vi "LV8_3.vi"() -> ()   [LabVIEW 2016]
uses:
  <vilib>/sound2/lvsound2.llb/Sampling Mode.ctl
  <vilib>/Utility/file.llb/Read From Spreadsheet File (DBL).vi
  <vilib>/imath/engines/lvmath2/RunTimeEngine/BuiltInFunctions/length/NIMS_length(GV).vi
  <instcachedir>/0/NIMS_length(GV)_08A3D13377FD4E4B96F5795FBF3698FA.lvgen/NIMS_length(GV)_08A3D13377FD4E4B96F5795FBF3698FA_000.vi
  <vilib>/imath/engines/lvmath2/RunTimeEngine/RangeToken/NIMS_Range.vi
  <instcachedir>/0/NIMS_Range_A7C094595B484CA7AF10685B02D808ED.lvgen/NIMS_Range_A7C094595B484CA7AF10685B02D808ED_001.vi
  <vilib>/imath/engines/lvmath2/RunTimeEngine/ArithmeticOperatorToken/NIMS_ArithmeticOperator_plus.vi
  <instcachedir>/0/NIMS_ArithmeticOperator_plus_0120E0498A0F4B4B9BDCAC2554767A4E.lvgen/NIMS_ArithmeticOperator_plus_0120E0498A0F4B4B9BDCAC2554767A4E_004.vi
  <vilib>/imath/engines/lvmath2/RunTimeEngine/ErrorHandling/NIMS_Create Error From Enums.vi
  <vilib>/imath/engines/lvmath2/RunTimeEngine/BuiltInFunctions/polyval/NIMS_polyval(GV,GM).vi
  <instcachedir>/0/NIMS_polyval(GV,GM)_E12556DC54744E0C81968744501C4F35.lvgen/NIMS_polyval(GV,GM)_E12556DC54744E0C81968744501C4F35_003.vi
  <vilib>/imath/engines/lvmath2/RunTimeEngine/ArithmeticOperatorToken/NIMS_ArithmeticOperator_rightdiv(C,C).vi
  <instcachedir>/0/NIMS_ArithmeticOperator_rightdiv(C,C)_6F3C2C239EC94040B0793F3E73F9E5CA.lvgen/NIMS_ArithmeticOperator_rightdiv(C,C)_6F3C2C239EC94040B0793F3E73F9E5CA_000.vi
  <vilib>/imathl/engines/lvmath/Functions/Error Handling/Create Error.vi
  <vilib>/imath/engines/lvmath2/RunTimeEngine/BuiltInFunctions/filter/NIMS_filter(GV,GV,GV,GV,Str).vi
  <instcachedir>/0/NIMS_filter(GV,GV,GV,GV,Str)_434E59EE96884CB3BC5141C85D3A0B2F.lvgen/NIMS_filter(GV,GV,GV,GV,Str)_434E59EE96884CB3BC5141C85D3A0B2F_000.vi
  <vilib>/imath/engines/lvmath2/RunTimeEngine/BuiltInFunctions/impzd/NIMS_impzd().vi
  <vilib>/imath/engines/lvmath2/RunTimeEngine/BuiltInFunctions/fft/NIMS_fft(GV).vi
  <instcachedir>/0/NIMS_fft(GV)_4C6467FC22F84E4BA42517A07EF978B0.lvgen/NIMS_fft(GV)_4C6467FC22F84E4BA42517A07EF978B0_000.vi
  <vilib>/imath/engines/lvmath2/RunTimeEngine/BuiltInFunctions/abs/NIMS_abs(signed).vi
  <instcachedir>/0/NIMS_abs(signed)_C4FCB8E6058B49B797C7C8D53CA5F6EC.lvgen/NIMS_abs(signed)_C4FCB8E6058B49B797C7C8D53CA5F6EC_006.vi
  <vilib>/imath/engines/lvmath2/RunTimeEngine/ErrorHandling/NIMS_Error From Error Code.vi
  <vilib>/imath/engines/lvmath2/RunTimeEngine/IndexRead/NIMS V(R2).vi
  <instcachedir>/0/NIMS V(R2)_C76619605A0E4E9F8B2FA9389712AC47.lvgen/NIMS V(R2)_C76619605A0E4E9F8B2FA9389712AC47_000.vi
  <vilib>/imath/engines/lvmath2/RunTimeEngine/NodeEndStatement/NIMS_NodeEndStatement_Output.vi
  <instcachedir>/0/NIMS_NodeEndStatement_Output_53EC0D466D134D7ABD903AC30B43404B.lvgen/NIMS_NodeEndStatement_Output_53EC0D466D134D7ABD903AC30B43404B_005.vi
  <instcachedir>/0/NIMS_NodeEndStatement_Output_53EC0D466D134D7ABD903AC30B43404B.lvgen/NIMS_NodeEndStatement_Output_53EC0D466D134D7ABD903AC30B43404B_000.vi
  <vilib>/imath/engines/lvmath2/RunTimeEngine/ErrorHandling/NIMS_Finalize Error.vi
  <vilib>/sound2/lvsound2.llb/Sound Output Write (DBL Single).vi
panel:
  in  "notch frequency":dbl(slide)=1500.0 scale=600.0..2000.0
  in  "pole radius":dbl(slide)=0.9 scale=0.5..0.99
  in  "Interference frequency":dbl(slide)=1500.0 scale=600.0..2000.0
  in  "Interference level":dbl(slide)=0.5 scale=0.0..1.0
  out "Filter impulse (time domain)":cluster{"t":dbl[], "h":dbl[]}(graph)={"t"=[0.0, 1.0, 2.0, 3.0, 4.0, 5.0, 6.0, 7.0, 8.0, 9.0, 10.0, 11.0, 12.0, 13.0, 14.0, 15.0, 16.0, 17.0, 18.0, 19.0, 20.0, 21.0, 22.0, 23.0, 24.0, 25.0, 26.0, 27.0, 28.0, 29.0, 30.0, 31.0, 32.0, 33.0, 34.0, 35.0, 36.0, 37.0, 38.0, 39.0, 40.0, 41.0, 42.0, 43.0, 44.0, 45.0, 46.0, 47.0, 48.0, 49.0, 50.0, 51.0, 52.0, 53.0, 54.0, 55.0, 56.0, 57.0, 58.0, 59.0, 60.0, 61.0, 62.0, 63.0, 64.0, 65.0, 66.0, 67.0, 68.0, 69.0, 70.0, 71.0, 72.0, 73.0, 74.0, 75.0, 76.0, 77.0, 78.0, 79.0, 80.0, 81.0, 82.0, 83.0, 84.0, 85.0, 86.0, 87.0, 88.0, 89.0, 90.0, 91.0, 92.0, 93.0, 94.0, 95.0, 96.0, 97.0, 98.0, 99.0], "h"=[1.0, -0.19544999929210816, -0.15380632000956734, -0.11223850680631889, -0.07285002547483177, -0.037233646334255716, -0.006487324712441719, 0.01874772503665746, 0.03823291862336755, 0.05206795798115917, 0.06062147707010433, 0.0644611628892075, 0.06428701174279264, 0.06087052565632748, 0.055001818256293536, 0.047445822271690086, 0.03890810057714032, 0.030010178032265383, 0.021273842008977223, 0.013113507444220199, 0.00583550315893764, -0.00035699923526721217, -0.005354737061261871, -0.009130080812930957, -0.011722931576196152, -0.013225857255946803, -0.013769369545092234, -0.013508065033252652, -0.01260817237915801, -0.011236872866296281, -0.009553601516750164, -0.007703395665473211, -0.005812240867704549, -0.003984271772272541, -0.0023006181327914123, -0.0008196421762888132, 0.0004217091225821308, 0.0014057175921853033, 0.0021311431322861706, 0.0026101560636003027, 0.0028651690698949664, 0.002925749222628381, 0.0028257522048094758, 0.0026007825275379793, 0.00228604720260032, 0.0019146374698639518, 0.0015162447950596892, 0.0011162940464999036, 0.0007354587513853615, 0.00038951053427375266, 8.944691421038304e-05, -0.00015816193888983356, -0.00035066675810689976, -0.0004887291881129679, -0.0005756590011697686, -0.0006167423199685475, -0.0006185967830638732, -0.000588581388132878, -0.0005342806927635217, -0.0004630755248140955, -0.0003818056378356512, -0.00029652402970290745, -0.00021233802591275242, -0.00013332873906976472, -6.25381166219509e-05, -2.0113949989798865e-06, 4.711773010347752e-05, 8.451167278747195e-05, 0.00011049489609454997, 0.0001259115913131821, 0.0001319839180606837, 0.00013017792126015324, 0.0001220824979341105, 0.00010930510099255216, 9.338631387780366e-05, 7.573406302784645e-05, 5.7577088845670426e-05, 3.993638671451698e-05, 2.3612658830734072e-05, 9.18737412711179e-06, -2.965203253235978e-06, -1.2657713806717492e-05, -1.9863736756039002e-05, -2.4688557830858333e-05, -2.7338780722664013e-05, -2.8092550212993024e-05, -2.7271787887851753e-05, -2.5217472637744435e-05, -2.2268646893473075e-05, -1.874551033941178e-05, -1.493668585922404e-05, -1.1090513790978811e-05, -7.410052667381395e-06, -4.051336926192118e-06, -1.1243615336631208e-06, 1.3037747615809595e-06, 3.204137828213956e-06, 4.5801810692416564e-06, 5.461415839630941e-06, 5.896956831399133e-06]}
  out "Signal + interference (freq)":cluster{"W":dbl[], "H":dbl[]}[](graph)
  out "Signal + interference (time domain)":cluster{"t":dbl[], "Y":dbl[]}(graph)={"t"=[0.0, 1.0, 2.0, 3.0, 4.0, 5.0, 6.0, 7.0, 8.0, 9.0, 10.0, 11.0, 12.0, 13.0, 14.0, 15.0, 16.0, 17.0, 18.0, 19.0, 20.0, 21.0, 22.0, 23.0, 24.0, 25.0, 26.0, 27.0, 28.0, 29.0, 30.0, 31.0, 32.0, 33.0, 34.0, 35.0, 36.0, 37.0, 38.0, 39.0, 40.0, 41.0, 42.0, 43.0, 44.0, 45.0, 46.0, 47.0, 48.0, 49.0, 50.0, 51.0, 52.0, 53.0, 54.0, 55.0, 56.0, 57.0, 58.0, 59.0, 60.0, 61.0, 62.0, 63.0, 64.0, 65.0, 66.0, 67.0, 68.0, 69.0, 70.0, 71.0, 72.0, 73.0, 74.0, 75.0, 76.0, 77.0, 78.0, 79.0, 80.0, 81.0, 82.0, 83.0, 84.0, 85.0, 86.0, 87.0, 88.0, 89.0, 90.0, 91.0, 92.0, 93.0, 94.0, 95.0, 96.0, 97.0, 98.0, 99.0], "Y"=array[32768 elements]}
  out "Filtered signal (freq domain)":cluster{"W":dbl[], "FZ":dbl[]}(graph)
  out "Original signal (freq domain)":cluster{"F":dbl[], "FXI":dbl[]}(graph)
  out "Original signal (time domain)":cluster{"t":dbl[], "first row":dbl[]}(graph)={"t"=[0.0, 1.0, 2.0, 3.0, 4.0, 5.0, 6.0, 7.0, 8.0, 9.0, 10.0, 11.0, 12.0, 13.0, 14.0, 15.0, 16.0, 17.0, 18.0, 19.0, 20.0, 21.0, 22.0, 23.0, 24.0, 25.0, 26.0, 27.0, 28.0, 29.0, 30.0, 31.0, 32.0, 33.0, 34.0, 35.0, 36.0, 37.0, 38.0, 39.0, 40.0, 41.0, 42.0, 43.0, 44.0, 45.0, 46.0, 47.0, 48.0, 49.0, 50.0, 51.0, 52.0, 53.0, 54.0, 55.0, 56.0, 57.0, 58.0, 59.0, 60.0, 61.0, 62.0, 63.0, 64.0, 65.0, 66.0, 67.0, 68.0, 69.0, 70.0, 71.0, 72.0, 73.0, 74.0, 75.0, 76.0, 77.0, 78.0, 79.0, 80.0, 81.0, 82.0, 83.0, 84.0, 85.0, 86.0, 87.0, 88.0, 89.0, 90.0, 91.0, 92.0, 93.0, 94.0, 95.0, 96.0, 97.0, 98.0, 99.0], "first row"=array[32768 elements]}
  out "Filtered signal (time domain)":cluster{"t":dbl[], "Z":dbl[]}(graph)={"t"=[0.0, 1.0, 2.0, 3.0, 4.0, 5.0, 6.0, 7.0, 8.0, 9.0, 10.0, 11.0, 12.0, 13.0, 14.0, 15.0, 16.0, 17.0, 18.0, 19.0, 20.0, 21.0, 22.0, 23.0, 24.0, 25.0, 26.0, 27.0, 28.0, 29.0, 30.0, 31.0, 32.0, 33.0, 34.0, 35.0, 36.0, 37.0, 38.0, 39.0, 40.0, 41.0, 42.0, 43.0, 44.0, 45.0, 46.0, 47.0, 48.0, 49.0, 50.0, 51.0, 52.0, 53.0, 54.0, 55.0, 56.0, 57.0, 58.0, 59.0, 60.0, 61.0, 62.0, 63.0, 64.0, 65.0, 66.0, 67.0, 68.0, 69.0, 70.0, 71.0, 72.0, 73.0, 74.0, 75.0, 76.0, 77.0, 78.0, 79.0, 80.0, 81.0, 82.0, 83.0, 84.0, 85.0, 86.0, 87.0, 88.0, 89.0, 90.0, 91.0, 92.0, 93.0, 94.0, 95.0, 96.0, 97.0, 98.0, 99.0], "Z"=array[32768 elements]}
  in  "Play original sound":bool
  in  "Play noisy sound":bool
  in  "Play filtered sound":bool
  in  "stop":bool
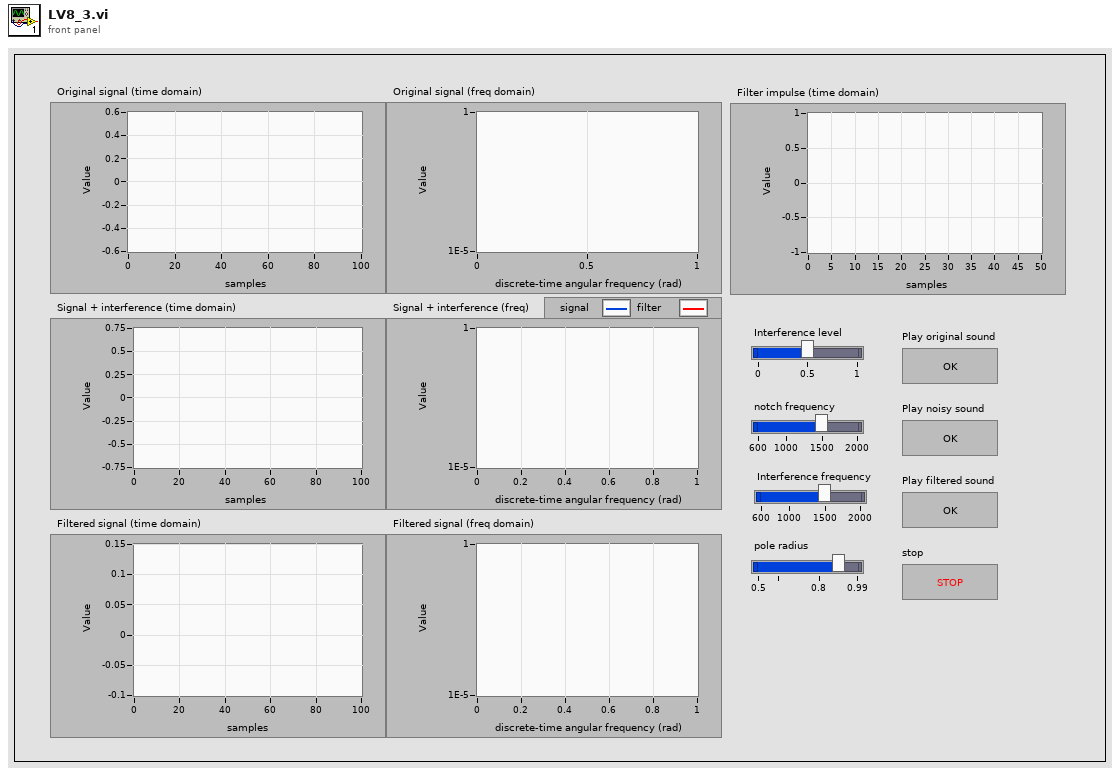
[diagram p1: front panel]
types:
  T1 = typedef "Sampling Mode.ctl" = i32
  T2 = typedef "Sound Output Task ID.ctl" = u32
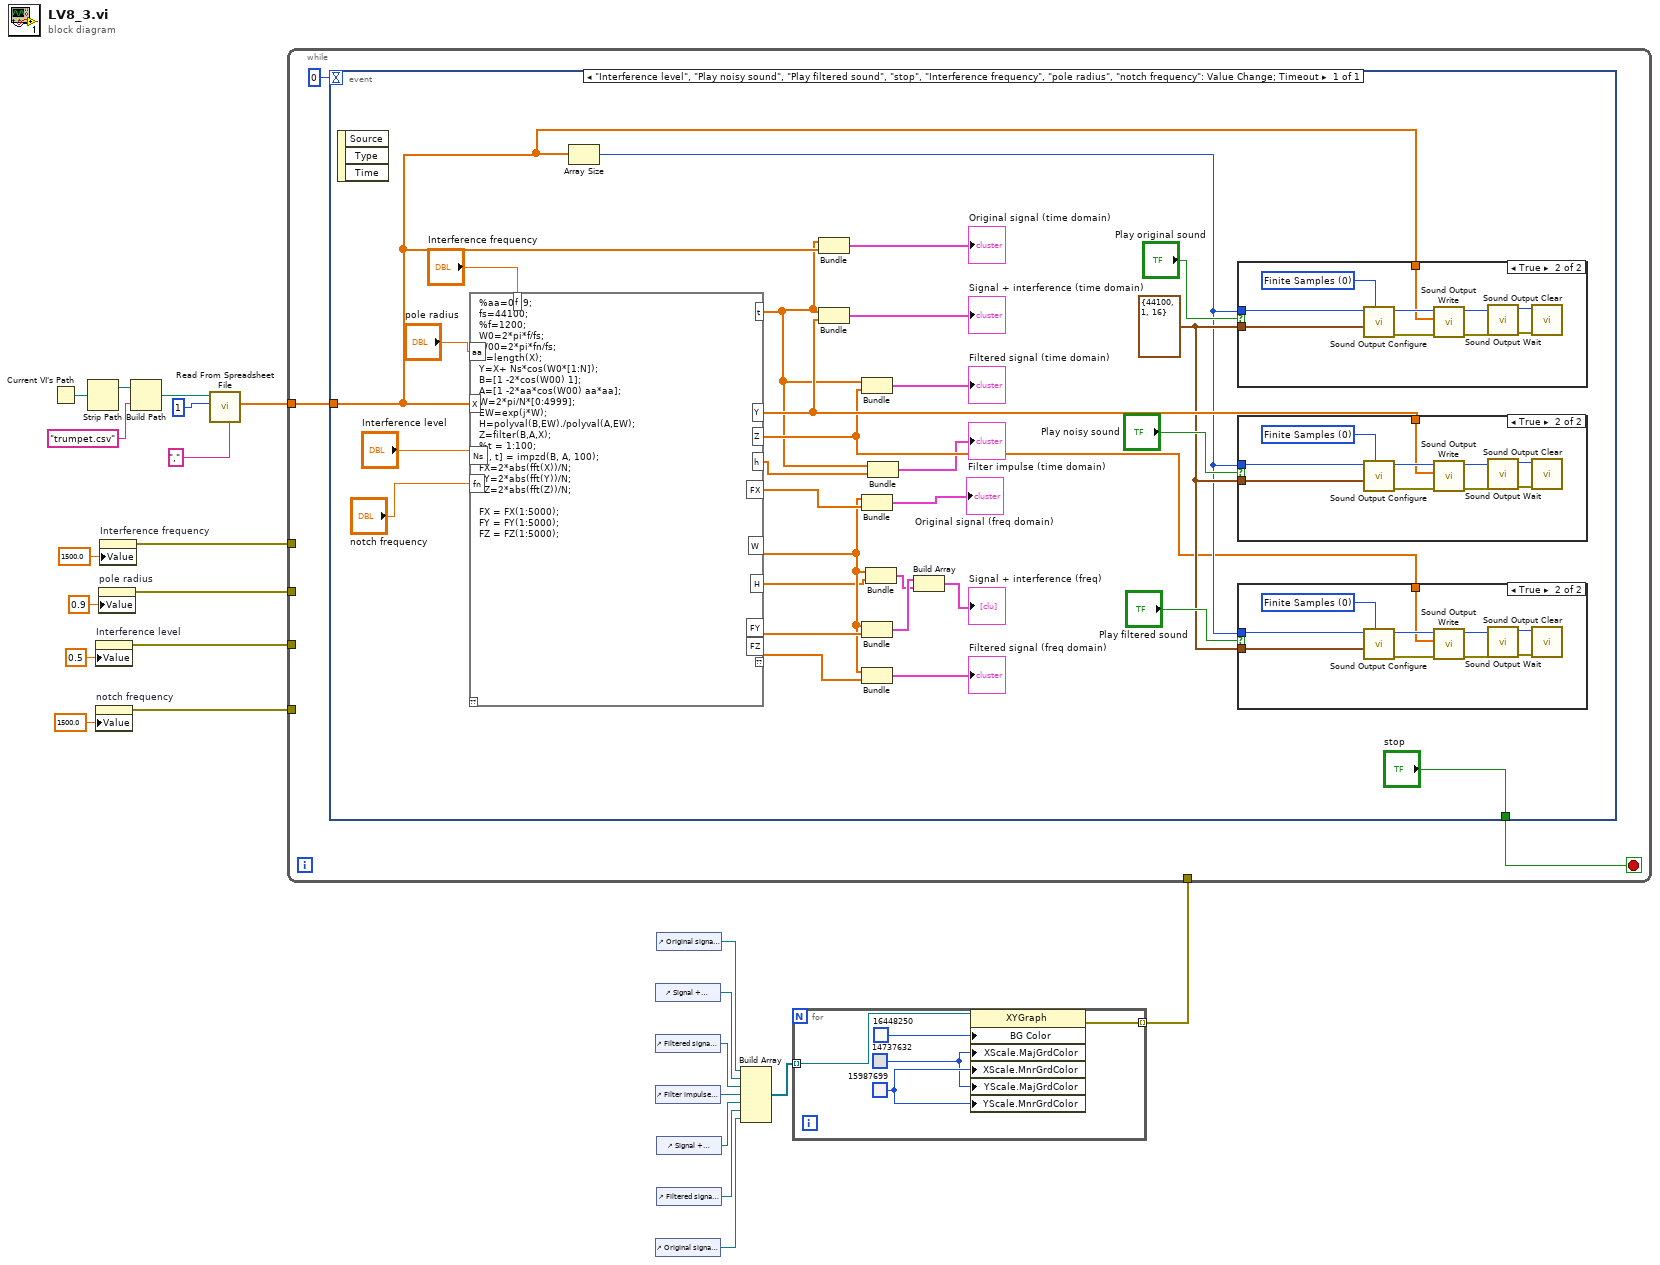
[diagram p0: block diagram]
diagram:
  n1 = Current VI's Path() -> (path=w24:path)
  n2 = Strip Path(path=w24) -> (stripped path=w23:path)  [unwired: 1 out]
  n3 = property on="Interference level" class="Slide (strict)"("Value"=0.5 ("Interference level")) -> (error out=w15:errorcluster)  [unwired: 2 in, 1 out]
  n4 = property on="notch frequency" class="Slide (strict)"("Value"=1500.0 ("notch frequency")) -> (error out=w11:errorcluster)  [unwired: 2 in, 1 out]
  n5 = property on="pole radius" class="Slide (strict)"("Value"=0.9 ("pole radius")) -> (error out=w16:errorcluster)  [unwired: 2 in, 1 out]
  n6 = property on="Interference frequency" class="Slide (strict)"("Value"=1500.0 ("Interference frequency")) -> (error out=w17:errorcluster)  [unwired: 2 in, 1 out]
  n7 = Build Path(base path=w23, name or relative path="trumpet.csv") -> (appended path=w21:path)
  n8 = call-poly <vilib>:"Read From Spreadsheet File.vi"("delimiter (\\t)"="," ("delimiter (\\t)"), "number of rows (all:-1)"=1, "file path (dialog if empty)"=w21) -> ("first row"=w18:dbl[])  [unwired: 4 in, 4 out]
  n9 = control-ref of="Signal + interference (time domain)"() -> (w6:refnum<vi>)
  n10 = control-ref of="Filtered signal (time domain)"() -> (w5:refnum<vi>)
  n11 = control-ref of="Filter impulse (time domain)"() -> (w4:refnum<vi>)
  n12 = control-ref of="Original signal (freq domain)"() -> (w1:refnum<vi>)
  n13 = control-ref of="Original signal (time domain)"() -> (w7:refnum<vi>)
  n14 = control-ref of="Signal + interference (freq)"() -> (w3:refnum<vi>)
  n15 = control-ref of="Filtered signal (freq domain)"() -> (w2:refnum<vi>)
  n16 = Build Array(w7, w6, w5, w4, w3, w2, w1) -> (w9:refnum<vi>[])
  n17 = for {
    tunnel: w9 -> [w26] mode=indexing
    tunnel: [w25] -> w8 mode=indexing
    w28 = u32 15987699
    w27 = u32 14737632
    n18 = property class="XYGraph"(reference=w26, "BG Color"=u32 16448250, "XScale.MajGrdColor"=w27, "XScale.MnrGrdColor"=w28, "YScale.MajGrdColor"=w27, "YScale.MnrGrdColor"=w28) -> (error out=w25:errorcluster)  [unwired: 1 in, 1 out]
  }
  n19 = while {
    tunnel: w18 -> [w32]
    tunnel: w17 -> [_]
    tunnel: w16 -> [_]
    tunnel: w15 -> [_]
    tunnel: w11 -> [_]
    tunnel: w8 -> [_]
    stop <- w31 stop-if-true
    n20 = event shown="[0] \"Interference level\", \"Play noisy sound\", \"Play filtered sound\", \"stop\", \"Interference frequency\", \"pole radius\", \"notch frequency\": Value Change;  Timeout" {
      selector: _ -> [_]
      dyn-events: _ -> [_]
      timeout: 0 -> [_]
      tunnel: w32 -> [w56]
      tunnel: ["stop"] -> w31
      event "Interference level", "Play noisy sound", "Play filtered sound", "stop", "Interference frequency", "pole radius", "notch frequency": Value Change; Timeout {
        w52 = cluster{"fs":i32, i32, i32} {"fs"=44100, 1, 16}
        n21 = event-data() -> ()  [unwired: 1 in, 3 out]
        n22 = mathscript code="%aa=0.99;\nfs=44100;\n%f=1200;\nW0=2*pi*f/fs;\nW00=2*pi*fn/fs;\nN=length(X);\nY=X+ Ns*cos(W0*[1:N]);\nB=[1 -2*cos(W00) 1];\nA=[1 -2*aa*cos(W00) aa*aa];\nW=2*pi/N*[0:4999];\nEW=exp(j*W);\nH=polyval(B,EW)./polyval(A,EW);\nZ=filter(B,A,X);\n%t = 1:100;\n[h, t] = impzd(B, A, 100);\nFX=2*abs(fft(X))/N;\nFY=2*abs(fft(Y))/N;\nFZ=2*abs(fft(Z))/N;\n\nFX = FX(1:5000);\nFY = FY(1:5000);\nFZ = FZ(1:5000);"("X"=w56, "aa"="pole radius", "Ns"="Interference level", "f"="Interference frequency", "fn"="notch frequency") -> ("Z"=w50:dbl[], "Y"=w54:dbl[], "W"=w45:dbl[], "FY"=w48:dbl[], "t"=w40:dbl[], "FZ"=w46:dbl[], "FX"=w47:dbl[], "H"=w41:cdb[], "h"=w39:dbl[])  [unwired: 1 in, 1 out]
        n23 = Array Size(array=w56) -> (size(s)=w51:i32)
        n24 = Bundle("t"=w40, "first row"=w56) -> (→"Original signal (time domain)":cluster{"t":dbl[], "first row":dbl[]})  [unwired: 1 in]
        n25 = Bundle("t"=w40, "Y"=w54) -> (→"Signal + interference (time domain)":cluster{"t":dbl[], "Y":dbl[]})  [unwired: 1 in]
        n26 = Bundle("t"=w40, "Z"=w50) -> (→"Filtered signal (time domain)":cluster{"t":dbl[], "Z":dbl[]})  [unwired: 1 in]
        n27 = Bundle("W"=w45, "FX"=w47) -> (→"Original signal (freq domain)":cluster{"W":dbl[], "FX":dbl[]})  [unwired: 1 in]
        n28 = Bundle("W"=w45, "FY"=w48) -> (w36:cluster{"W":dbl[], "FY":dbl[]})  [unwired: 1 in]
        n29 = Bundle("W"=w45, "FZ"=w46) -> (→"Filtered signal (freq domain)":cluster{"W":dbl[], "FZ":dbl[]})  [unwired: 1 in]
        n30 = Bundle("W"=w45, "H"=w41) -> (w35:cluster{"W":dbl[], "H":cdb[]})  [unwired: 1 in]
        n31 = Bundle("t"=w40, "h"=w39) -> (→"Filter impulse (time domain)":cluster{"t":dbl[], "h":dbl[]})  [unwired: 1 in]
        n32 = Build Array(w36, w35) -> (→"Signal + interference (freq)":cluster{"W":dbl[], "H":cdb[]}[])
        n33 = case shown="True" "Play original sound" {
          tunnel: w52 -> [_ w437]
          tunnel: w51 -> [_ w435]
          tunnel: w56 -> [_ w434]
          frame False {
          }
          frame True {
            w436 = T1 0 items=["Finite Samples", "Continuous Samples"] ("sample mode")
            n34 = call <vilib>:"Sound Output Configure.vi"("number of samples/ch"=w435, "sample mode"=w436, "sound format"=w437) -> ("error out"=w438:errorcluster, "task ID"=w443:T2)  [unwired: 7 in]
            n35 = call-poly <vilib>:"Sound Output Write.vi"("error in (no error)"=w438, "data"=w434, "task ID"=w443) -> ("error out"=w439:errorcluster, "task ID out"=w440:T2)  [unwired: 7 in]
            n36 = call <vilib>:"Sound Output Wait.vi"("error in (no error)"=w439, "task ID"=w440) -> ("error out"=w442:errorcluster, "task ID out"=w441:T2)  [unwired: 8 in]
            n37 = call <vilib>:"Sound Output Clear.vi"("error in (no error)"=w442, "task ID"=w441) -> ()  [unwired: 9 in, 1 out]
          }
        }
        n38 = case shown="True" "Play noisy sound" {
          tunnel: w52 -> [_ w427]
          tunnel: w51 -> [_ w425]
          tunnel: w54 -> [_ w424]
          frame False {
          }
          frame True {
            w426 = T1 0 items=["Finite Samples", "Continuous Samples"] ("sample mode")
            n39 = call <vilib>:"Sound Output Configure.vi"("number of samples/ch"=w425, "sample mode"=w426, "sound format"=w427) -> ("error out"=w428:errorcluster, "task ID"=w433:T2)  [unwired: 7 in]
            n40 = call-poly <vilib>:"Sound Output Write.vi"("error in (no error)"=w428, "data"=w424, "task ID"=w433) -> ("error out"=w429:errorcluster, "task ID out"=w430:T2)  [unwired: 7 in]
            n41 = call <vilib>:"Sound Output Wait.vi"("error in (no error)"=w429, "task ID"=w430) -> ("error out"=w432:errorcluster, "task ID out"=w431:T2)  [unwired: 8 in]
            n42 = call <vilib>:"Sound Output Clear.vi"("error in (no error)"=w432, "task ID"=w431) -> ()  [unwired: 9 in, 1 out]
          }
        }
        n43 = case shown="True" "Play filtered sound" {
          tunnel: w52 -> [_ w417]
          tunnel: w51 -> [_ w415]
          tunnel: w50 -> [_ w414]
          frame False {
          }
          frame True {
            w416 = T1 0 items=["Finite Samples", "Continuous Samples"] ("sample mode")
            n44 = call <vilib>:"Sound Output Configure.vi"("number of samples/ch"=w415, "sample mode"=w416, "sound format"=w417) -> ("error out"=w418:errorcluster, "task ID"=w423:T2)  [unwired: 7 in]
            n45 = call-poly <vilib>:"Sound Output Write.vi"("error in (no error)"=w418, "data"=w414, "task ID"=w423) -> ("error out"=w419:errorcluster, "task ID out"=w420:T2)  [unwired: 7 in]
            n46 = call <vilib>:"Sound Output Wait.vi"("error in (no error)"=w419, "task ID"=w420) -> ("error out"=w422:errorcluster, "task ID out"=w421:T2)  [unwired: 8 in]
            n47 = call <vilib>:"Sound Output Clear.vi"("error in (no error)"=w422, "task ID"=w421) -> ()  [unwired: 9 in, 1 out]
          }
        }
      }
    }
  }
